vi "Add Text.vi"(5 "Adr":string, 7 "Index":i32, 8 "error in":errorcluster, 10 "text":string, 11 "XLS in":refnum<class "XLS.lvclass">=refnum) -> (0 "error out":errorcluster, 3 "XLS out":refnum<class "XLS.lvclass">)   [LabVIEW 2017, in "Report_lib.lvlib" / "XLS.lvclass"]
doc: "This method Add the text\nto the xls report on previously\ndefined Coordinates"
uses:
  XLS.lvclass
  <vilib>/Utility/NIReport.llb/NI_report.lvclass
  <vilib>/Utility/NIReport.llb/Append Report Text (str wrap).vi
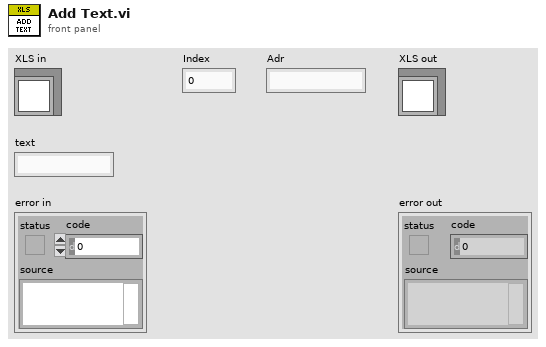
[diagram p1: front panel]
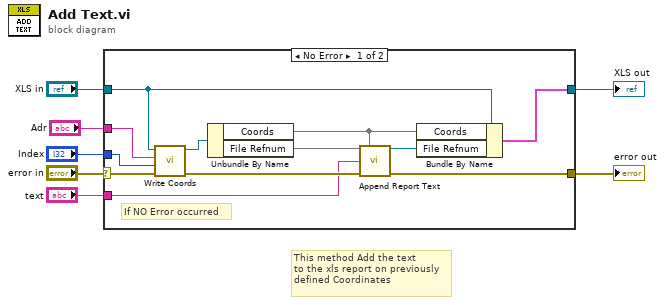
[diagram p0: block diagram]
diagram:
  # "This method Add the text\nto the xls report on previously\ndefined Coordinates"
  n1 = case shown="No Error" "error in" {
    selector: "error in" -> [w13 w21]
    tunnel: [w18 w21] -> w6
    tunnel: [w16 w20] -> w4
    tunnel: "XLS in" -> [w15 w20]
    tunnel: "text" -> [w11 _]
    tunnel: "Adr" -> [w10 _]
    tunnel: "Index" -> [w9 _]
    frame No Error {
      # "If NO Error occurred"
      n2 = call "Write Coords.vi"("error in"=w13, "Index"=w9, "Adr"=w10, "XLS in"=w15) -> ("error out"=w12:errorcluster, "XLS out"=w14:refnum<class "XLS.lvclass">)  [unwired: 6 in]
      n3 = Unbundle By Name(w14) -> ("Coords"=w8, "File Refnum"=w19)
      n4 = call-poly <vilib>:"Append Report Text.vi"("report in"=w19, "MS Office parameters"=w8, "text"=w11, "error in (no error)"=w12) -> ("report out"=w17:refnum<class "NI_report.lvclass">, "error out"=w18:errorcluster)  [unwired: 8 in, 2 out]
      n5 = Bundle By Name(cluster=w15, "Coords"=w8, "File Refnum"=w17) -> (w16:cluster{})
    }
    frame Error {
    }
  }
  "error out" <- w6
  "XLS out" <- w4
